vi "Memory.Pointer.Check.Offset.vi"(10 "offset in":u64 format="%d bytes", 11 "Pointer in":refnum<class "Memory.Pointer.lvclass">) -> (1 "valid offset?":bool, 2 "offset out":u64 format="%d bytes", 3 "Pointer out":refnum<class "Memory.Pointer.lvclass">)   [LabVIEW 2016, in "Memory.lvlib" / "Memory.Pointer.lvclass"]
uses:
  Memory.Pointer.lvclass
  Memory.Pointer.lvclass/Memory.Pointer.ctl
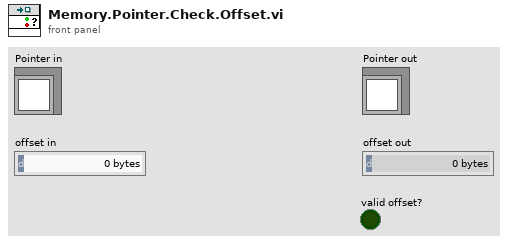
[diagram p1: front panel]
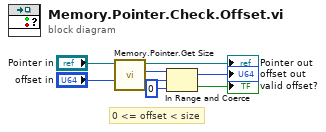
[diagram p0: block diagram]
diagram:
  # "0 <= offset < size"
  n1 = call "Memory.Pointer.Get Size.vi"("Pointer in"="Pointer in") -> ("size"=w5:u64, "Pointer out"=→"Pointer out":refnum<class "Memory.Pointer.lvclass">)  [unwired: 9 in]
  n2 = In Range and Coerce(upper limit=w5, x="offset in", lower limit=u64 0) -> (coerced(x)=→"offset out":u64, In Range?=→"valid offset?":bool)
